vi "Test Switches Module API.vi"() -> ()   [LabVIEW 2018]
doc: "Switches Module API Tester."
uses:
  MB switches Module.lvlib
panel:
  in  "mux2-1(DMM I) encode":enum16{"DMM I (0.5)", "DMM I (12)"}(ring)
  in  "DMM I 0.5_10":bool
  in  "mux6_1(3wires)_encode":T1(ring)
  in  "inst.mux6_1(3wires)":bool
  in  "mux10_1(x6)_encode":T2(ring)
  in  "inst.mux10_1":bool
  out "Optos":bool[](array[boolean])
  in  "Read Optos":bool
  in  "inst.Close":bool
  in  "VISA resource name":refnum<visa-resource-name>="COM11"
  in  "inst.Open":bool
  out "internal Counter":u16
  in  "Read Counter":bool
  in  "wait for reply":bool=TRUE
  in  "Show Block Diagram":bool
  in  "X":dbl=1.0
  out "Reply Payload":dbl
  in  "Stop Module":bool
  in  "Start Module":bool
  in  "Test Do Something Else and Wait for Reply":bool
  in  "Hide Module Panel":bool
  in  "Show Module Panel":bool
  in  "Test Do Something Else":bool
  in  "Test Do Something":bool
  out "Status":string
  out "Module Running?":bool
  # "This VI tests the API for the Module."
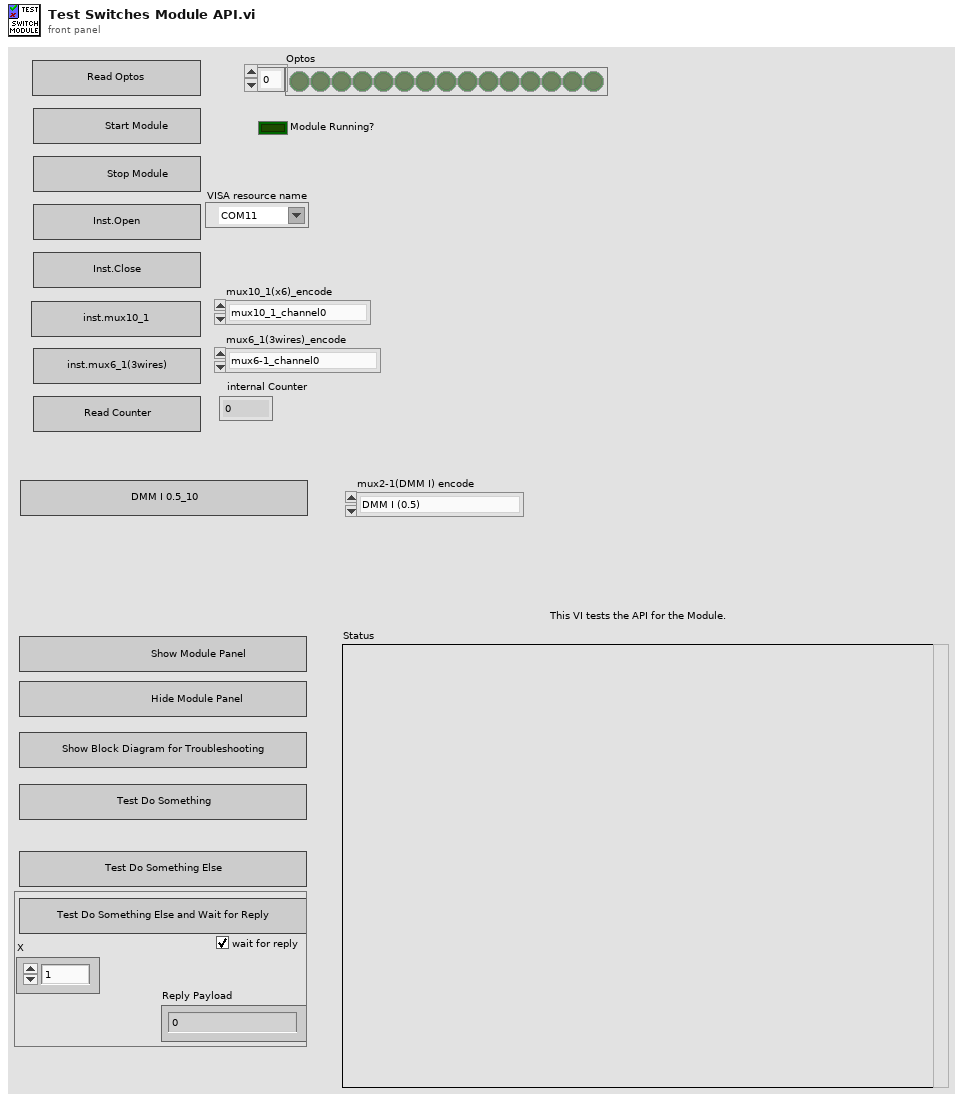
[diagram p1: front panel]
types:
  T1 = enum16{"mux6-1_channel0", "mux6_1_channel1_0", "mux6_1_channel1_1", "mux6-1_channel1_2", "mux6_1_channel1_3", "mux6_1_channel2_0", "mux6_1_channel2_1", "mux6_1_channel2_2", "mux6_1_channel2_3", "mux6_1_channel3_0", "mux6_1_channel3_1", "mux6_1_channel3_2", "mux6_1_channel3_3", "mux6_1_channel4_0", "mux6_1_channel4_1", "mux6_1_channel4_2", "mux6_1_channel4_3", "mux6_1_channel5_0", "mux6_1_channel5_1", "mux6_1_channel5_2", "mux6_1_channel5_3", "mux6_1_channel6_0", "mux6_1_channel6_1", "mux6_1_channel6_2", "mux6_1_channel6_3"}
  T2 = enum16{"mux10_1_channel0", "mux10_1_channel1", "mux10_1_channel2", "mux10_1_channel3", "mux10_1_channel4", "mux10_1_channel5", "mux10_1_channel6", "mux10_1_channel7", "mux10_1_channel8", "mux10_1_channel9", "mux10_1_channel10"}
  T3 = typedef "MB switches Module.lvlib/Broadcast Events--cluster.ctl" = cluster{"Module Did Init":refnum<user-event>, "Status Updated":refnum<user-event>, "Error Reported":refnum<user-event>, "Module Did Stop":refnum<user-event>, "Update Module Execution Status":refnum<user-event>}
  T4 = typedef "MB switches Module.lvlib/Do Something Else and Wait (Reply Payload)--cluster.ctl" = cluster{"Value":dbl, "error":errorcluster}
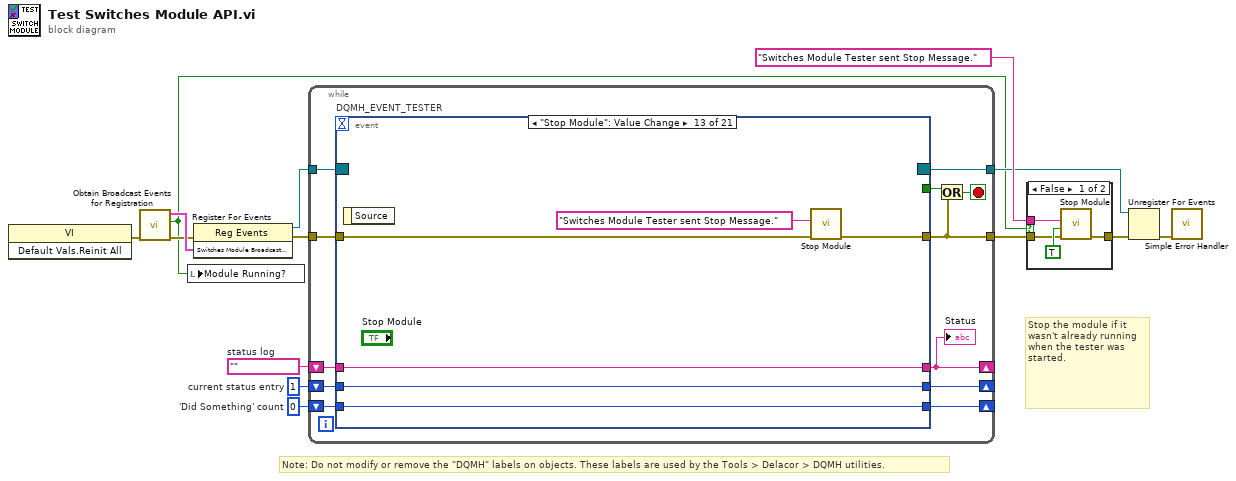
[diagram p0: block diagram]
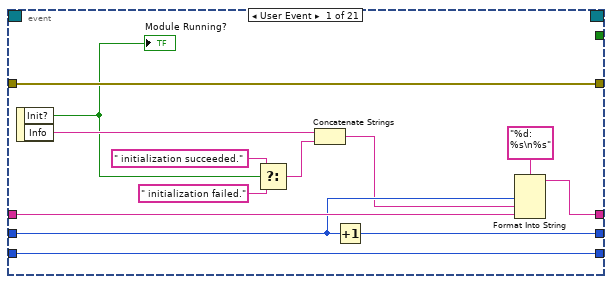
[diagram p3: hidden frame]
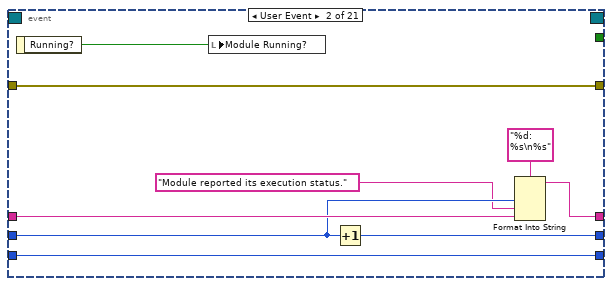
[diagram p4: hidden frame]
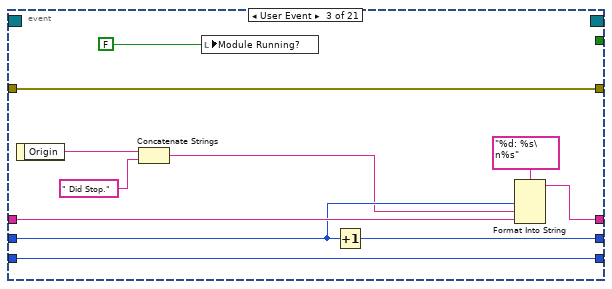
[diagram p5: hidden frame]
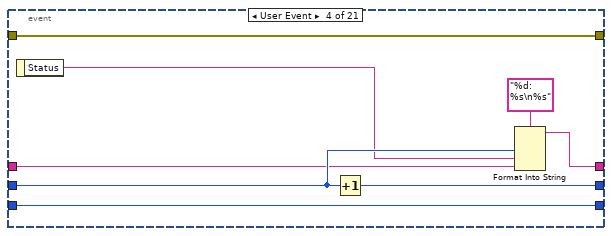
[diagram p6: hidden frame]
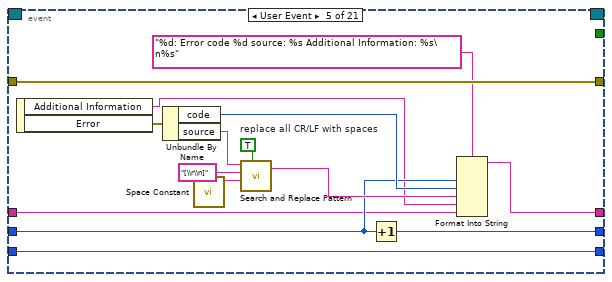
[diagram p7: hidden frame]
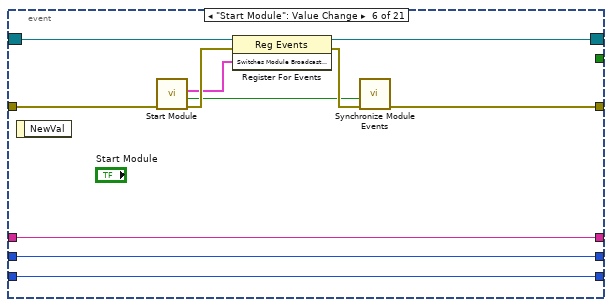
[diagram p8: hidden frame]
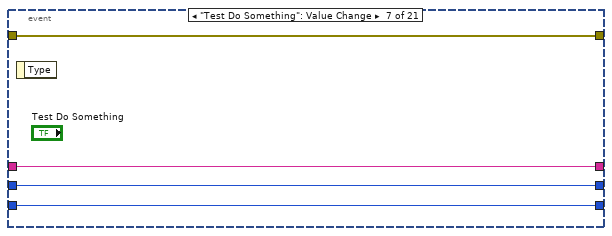
[diagram p9: hidden frame]
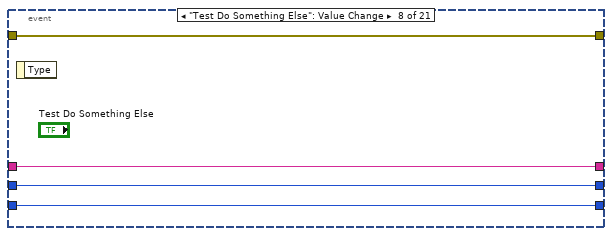
[diagram p10: hidden frame]
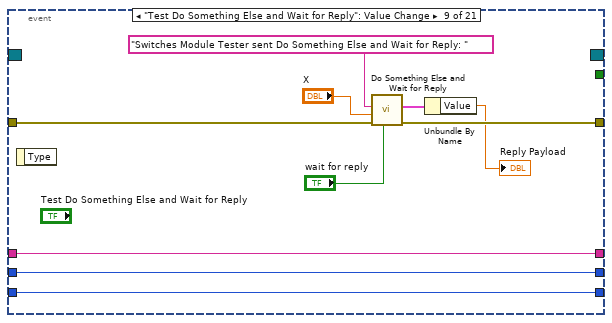
[diagram p11: hidden frame]
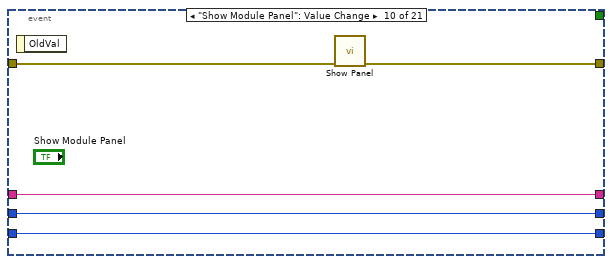
[diagram p12: hidden frame]
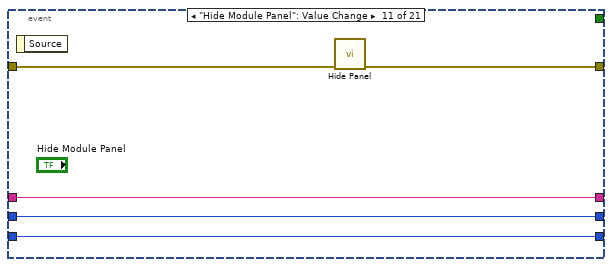
[diagram p13: hidden frame]
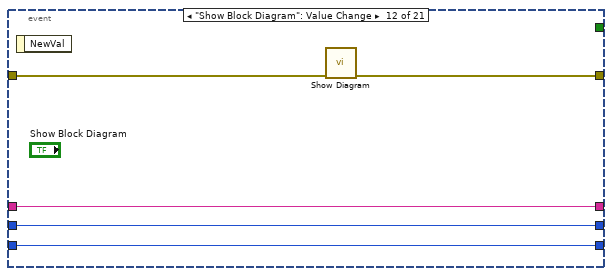
[diagram p14: hidden frame]
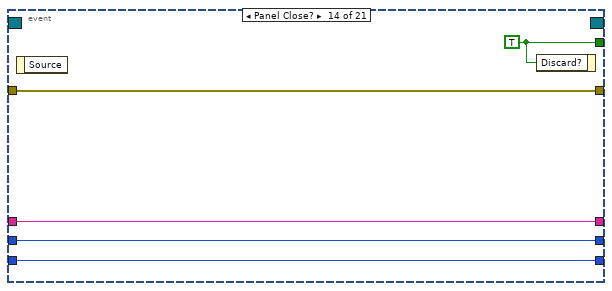
[diagram p15: hidden frame]
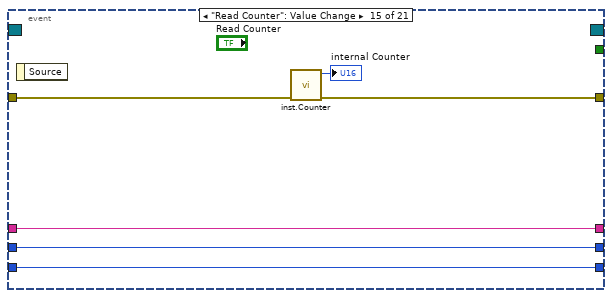
[diagram p16: hidden frame]
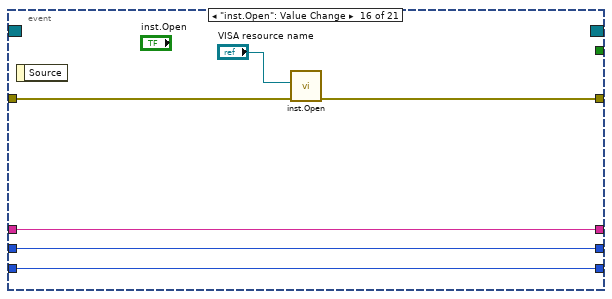
[diagram p17: hidden frame]
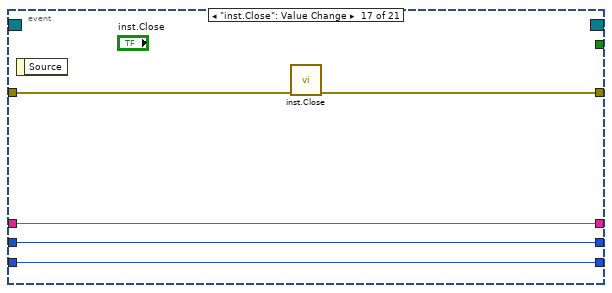
[diagram p18: hidden frame]
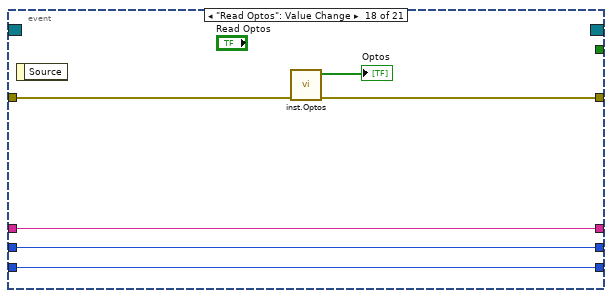
[diagram p19: hidden frame]
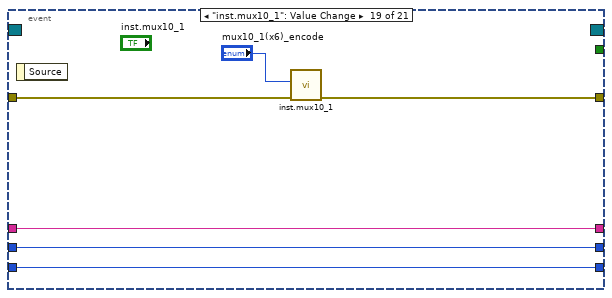
[diagram p20: hidden frame]
diagram:
  w10 = 0  # 'Did Something' count
  w11 = 1  # current status entry
  w12 = ""  # status log
  # "Stop the module if it wasn't already running when the tester was started."
  # "Note: Do not modify or remove the \"DQMH\" labels on objects. These labels are used by the Tools > Delacor > DQMH utilities."
  n1 = invoke class="VI" method="Default Vals.Reinit All"() -> (error out=w5:errorcluster)  [unwired: 3 in, 2 out]
  n2 = call "Obtain Broadcast Events for Registration.vi"("error in (no error)"=w5) -> ("error out"=w4:errorcluster, "Already running?"=w3:bool, "Switches Module Broadcast Events"=w8:T3)  [unwired: 8 in]
  n3 = local write "Module Running?"(w3) -> ()
  n4 = register-events(error in=w4, w8) -> (reference out=w7:refnum<event-registration>, error out=w9:errorcluster)  [unwired: 1 in]
  n5 = while {
    tunnel: w7 -> [w26]
    tunnel: [w15] -> w2
    shift-right: [w21] -> _
    shift-left: w12 -> [w23]
    shift-right: [w22] -> _
    shift-left: w11 -> [w24]
    shift-right: [w19] -> _
    shift-left: w10 -> [w20]
    tunnel: w9 -> [w17]
    tunnel: [w16] -> w6
    stop <- w18 stop-if-true
    n6 = event "DQMH_EVENT_TESTER" shown="[12] \"Stop Module\": Value Change" {
      selector: w26 -> [_ _ _ _ _ w86 _ _ _ _ _ _ _ _ _ _ _ _ _ _ _]
      dyn-events: [_ _ _ _ _ w85 _ _ _ _ _ _ _ _ _ _ _ _ _ _ _] -> w16
      timeout: _ -> [_ _ _ _ _ _ _ _ _ _ _ _ _ _ _ _ _ _ _ _ _]
      tunnel: [_ _ _ _ _ _ _ _ _ _ _ _ _ w137 _ _ _ _ _ _ _] -> w25
      tunnel: [w39 w41 w49 w60 w81 w84 w94 w98 w111 w116 w121 w122 w129 w133 w139 w145 w150 w156 w162 w168 w174] -> w15
      tunnel: w24 -> [w36 w46 w57 w64 w71 w90 w96 w100 w108 w114 w119 w124 w131 w135 w141 w147 w152 w158 w164 w170 w176]
      tunnel: w23 -> [w37 w47 w58 w63 w69 w91 w97 w101 w109 w115 w120 w125 w132 w136 w142 w148 w153 w159 w165 w171 w177]
      tunnel: [w34 w44 w55 w65 w72 w91 w97 w101 w109 w115 w120 w125 w132 w136 w142 w148 w153 w159 w165 w171 w177] -> w21
      tunnel: [w35 w45 w56 w67 w70 w90 w96 w100 w108 w114 w119 w124 w131 w135 w141 w147 w152 w158 w164 w170 w176] -> w22
      tunnel: w20 -> [w31 w42 w51 w61 w82 w89 w95 w99 w107 w113 w118 w123 w130 w134 w140 w146 w151 w157 w163 w169 w175]
      tunnel: [w31 w42 w51 w61 w82 w89 w95 w99 w107 w113 w118 w123 w130 w134 w140 w146 w151 w157 w163 w169 w175] -> w19
      tunnel: w17 -> [w39 w41 w49 w60 w81 w83 w94 w98 w104 w112 w117 w126 w127 w133 w143 w149 w154 w160 w166 w172 w178]
      event User Event {
        n7 = event-data() -> ("Init?"=w30:bool, "Info"=w33:string)  [unwired: 1 in]
        "Module Running?" <- w30
        n8 = Select(t=" initialization succeeded.", s=w30, f=" initialization failed.") -> (s? t:f=w27:string)
        n9 = Concatenate Strings(w33, w27) -> (w32:string)
        n10 = Increment(x=w36) -> (x+1=w35:i32)
        n11 = Format Into String(format string="%d: %s\n%s", w36, w32, w37) -> (resulting string=w34:string)  [unwired: 2 in, 1 out]
      }
      event User Event {
        n12 = event-data() -> ("Running?"=w40:bool)  [unwired: 1 in]
        n13 = local write "Module Running?"(w40) -> ()
        n14 = Increment(x=w46) -> (x+1=w45:i32)
        n15 = Format Into String(format string="%d: %s\n%s", w46, "Module reported its execution status.", w47) -> (resulting string=w44:string)  [unwired: 2 in, 1 out]
      }
      event User Event {
        n16 = event-data() -> ("Origin"=w54:string)  [unwired: 1 in]
        n17 = Concatenate Strings(w54, " Did Stop.") -> (w53:string)
        n18 = local write "Module Running?"(FALSE ("Module Did Init?")) -> ()
        n19 = Increment(x=w57) -> (x+1=w56:i32)
        n20 = Format Into String(format string="%d: %s\n%s", w57, w53, w58) -> (resulting string=w55:string)  [unwired: 2 in, 1 out]
      }
      event User Event {
        n21 = event-data() -> ("Status"=w62:string)  [unwired: 1 in]
        n22 = Increment(x=w64) -> (x+1=w67:i32)
        n23 = Format Into String(format string="%d: %s\n%s", w64, w62, w63) -> (resulting string=w65:string)  [unwired: 2 in, 1 out]
      }
      event User Event {
        w77 = TRUE  # replace all CR/LF with spaces
        n24 = event-data() -> ("Additional Information"=w68:string, "Error"=w73:errorcluster)  [unwired: 1 in]
        n25 = Unbundle By Name(w73) -> ("code"=w74:i32, "source"=w75:string)
        n26 = call <vilib>:"Space Constant.vi"() -> ("String"=w78:string)
        n27 = call <vilib>:"Search and Replace Pattern.vi"("string"=w75, "regular expression (\"\")"="[\\r\\n]" ("regular expression (\"\")"), "replace string (\"\")"=w78, "replace all? (F)"=w77) -> ("result string"=w76:string)  [unwired: 1 in, 1 out]
        n28 = Increment(x=w71) -> (x+1=w70:i32)
        n29 = Format Into String(format string="%d: Error code %d source: %s Additional Information: %s\n%s", w71, w74, w76, w68, w69) -> (resulting string=w72:string)  [unwired: 2 in, 1 out]
      }
      event "Start Module": Value Change {
        n30 = event-data() -> ()  [unwired: 1 in, 1 out]
        n31 = call "Start Module.vi"("error in (no error)"=w83) -> ("error out"=w92:errorcluster, "Wait for Event Sync?"=w88:bool, "Switches Module Broadcast Events"=w87:T3)  [unwired: 7 in, 1 out]
        n32 = register-events(reference=w86, error in=w92, w87) -> (reference out=w85:refnum<event-registration>, error out=w93:errorcluster)
        n33 = call "Synchronize Module Events.vi"("error in"=w93, "Wait for Event Sync?"=w88) -> ("error out"=w84:errorcluster)  [unwired: 9 in]
      }
      event "Test Do Something": Value Change {
        n34 = event-data() -> ()  [unwired: 1 in, 1 out]
      }
      event "Test Do Something Else": Value Change {
        n35 = event-data() -> ()  [unwired: 1 in, 1 out]
      }
      event "Test Do Something Else and Wait for Reply": Value Change {
        n36 = event-data() -> ()  [unwired: 1 in, 1 out]
        n37 = call "Do Something Else and Wait for Reply.vi"("wait for reply (T)"="wait for reply", "error in (no error)"=w104, "X"="X", "Do Something Else Message"="Switches Module Tester sent Do Something Else and Wait for Reply: " ("Do Something Message")) -> ("error out"=w111:errorcluster, "Reply Payload"=w106:T4)  [unwired: 5 in, 1 out]
        n38 = Unbundle By Name(w106) -> ("Value"=→"Reply Payload":dbl)
      }
      event "Show Module Panel": Value Change {
        n39 = event-data() -> ()  [unwired: 1 in, 1 out]
        n40 = call "Show Panel.vi"("error in (no error)"=w112) -> ("error out"=w116:errorcluster)  [unwired: 10 in]
      }
      event "Hide Module Panel": Value Change {
        n41 = event-data() -> ()  [unwired: 1 in, 1 out]
        n42 = call "Hide Panel.vi"("error in (no error)"=w117) -> ("error out"=w121:errorcluster)  [unwired: 10 in]
      }
      event "Show Block Diagram": Value Change {
        n43 = event-data() -> ()  [unwired: 1 in, 1 out]
        n44 = call "Show Diagram.vi"("error in (no error)"=w126) -> ("error out"=w122:errorcluster)  [unwired: 10 in]
      }
      event "Stop Module": Value Change {
        n45 = event-data() -> ()  [unwired: 1 in, 1 out]
        n46 = call "Stop Module.vi"("error in"=w127, "Origin"="Switches Module Tester sent Stop Message.") -> ("error out"=w129:errorcluster)  [unwired: 9 in]
      }
      event Panel Close? {
        w137 = TRUE ("Discard?")
        n47 = event-data() -> ()  [unwired: 1 in, 1 out]
        n48 = event-data("Discard?"=w137) -> ()  [unwired: 1 in, 1 out]
      }
      event "Read Counter": Value Change {
        n49 = event-data() -> ()  [unwired: 1 in, 1 out]
        n50 = call "inst.Counter.vi"("error in"=w143) -> ("error out"=w139:errorcluster, "counter"=→"internal Counter":u16)  [unwired: 8 in, 1 out]
      }
      event "inst.Open": Value Change {
        n51 = event-data() -> ()  [unwired: 1 in, 1 out]
        n52 = call "inst.Open.vi"("error in"=w149, "VISA resource name"="VISA resource name") -> ("error out"=w145:errorcluster)  [unwired: 9 in]
      }
      event "inst.Close": Value Change {
        n53 = event-data() -> ()  [unwired: 1 in, 1 out]
        n54 = call "inst.Close.vi"("error in"=w154) -> ("error out"=w150:errorcluster)  [unwired: 10 in]
      }
      event "Read Optos": Value Change {
        n55 = event-data() -> ()  [unwired: 1 in, 1 out]
        n56 = call "inst.Optos.vi"("error in"=w160) -> ("error out"=w156:errorcluster, "Optos"=→"Optos":bool[])  [unwired: 8 in, 1 out]
      }
      event "inst.mux10_1": Value Change {
        n57 = event-data() -> ()  [unwired: 1 in, 1 out]
        n58 = call "inst.mux10_1.vi"("error in"=w166, "mux10_1(x6)_encode"="mux10_1(x6)_encode") -> ("error out"=w162:errorcluster)  [unwired: 9 in]
      }
      event "mux6_1(3wires)_encode": Value Change {
        n59 = event-data() -> ()  [unwired: 1 in, 1 out]
        n60 = call "inst.mux6_1(3wires).vi"("error in"=w172, "mux6_1(3wires)_encode"="mux6_1(3wires)_encode") -> ("error out"=w168:errorcluster)  [unwired: 9 in]
      }
      event "DMM I 0.5_10": Value Change {
        n61 = event-data() -> ()  [unwired: 1 in, 1 out]
        n62 = call "DMM I 0.5_10.vi"("error in"=w178, "mux2-1(DMM I) encode"="mux2-1(DMM I) encode") -> ("error out"=w174:errorcluster)  [unwired: 9 in]
      }
    }
    "Status" <- w21
    n63 = Or(x=w25, y=w15) -> (x .or. y?=w18:bool)
  }
  n64 = case shown="False" w3 {
    tunnel: [w182 w183] -> w14
    tunnel: "Switches Module Tester sent Stop Message." ("Origin") -> [w181 _]
    tunnel: w2 -> [w179 w183]
    frame False {
      n65 = call "Stop Module.vi"("error in"=w179, "Wait for Module to Stop? (F)"=TRUE ("Wait for Module to stop?"), "Origin"=w181) -> ("error out"=w182:errorcluster)  [unwired: 8 in]
    }
    frame True {
    }
  }
  n66 = Unregister For Events(event registration refnum=w6, error in=w14) -> (error out=w1:errorcluster)
  n67 = call <vilib>:"Simple Error Handler.vi"("error in (no error)"=w1) -> ()  [unwired: 4 in, 5 out]
